vi "ProdaNG.Oracle.FindPath.vi"(8 "error in (no error)":errorcluster) -> (0 "error out":errorcluster, 1 "found":bool, 2 "Tnsnames path":path)   [LabVIEW 2016]
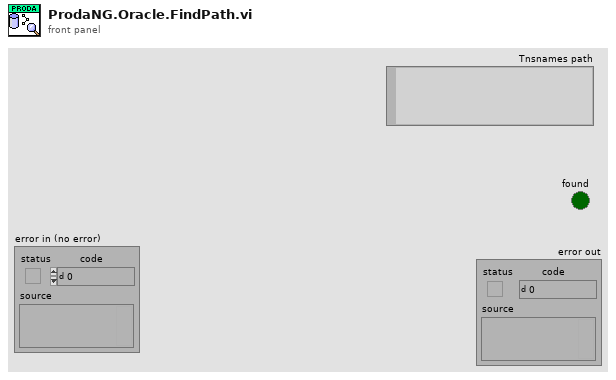
[diagram p1: front panel]
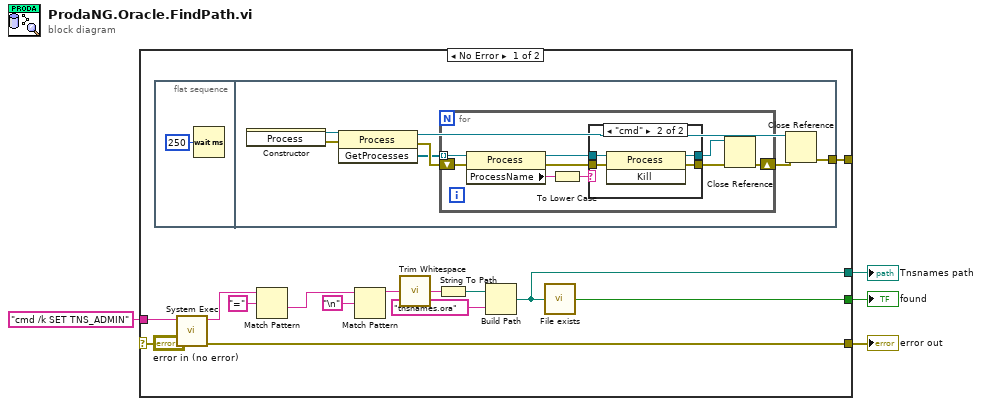
[diagram p0: block diagram]
diagram:
  n1 = case shown="No Error" "error in (no error)" {
    selector: "error in (no error)" -> [w18 w43]
    tunnel: "cmd /k SET TNS_ADMIN" ("command line") -> [w19 _]
    tunnel: [w17 w43] -> w4
    tunnel: [w11 _] -> w2
    tunnel: [w10 _] -> w1
    tunnel: [w6 _] -> _
    frame No Error {
      n2 = flat-sequence {
        tunnel: [w21] -> w6
        frame #0 {
          n3 = Wait (ms)(milliseconds to wait=u32 250) -> ()  [unwired: 1 out]
        }
        frame #1 {
          n4 = constructor class="Process"() -> (reference out=w27:refnum<k24>, error out=w26:errorcluster)  [unwired: 3 in, 1 out]
          n5 = invoke class="Process" method="GetProcesses"(reference=w27, error in=w26) -> (reference out=w22:refnum<k24>, error out=w25:errorcluster, "GetProcesses"=w24:refnum<k24>[])  [unwired: 1 in]
          n6 = for {
            tunnel: w24 -> [w36] mode=indexing
            shift-right: [w30] -> w23
            shift-left: w25 -> [w35]
            n7 = property class="Process"(reference=w36, error in=w35) -> (reference out=w34:refnum<k24>, error out=w33:errorcluster, "ProcessName"=w29:string)
            n8 = To Lower Case(string=w29) -> (all lower case string=w28:string)
            n9 = case shown="\"cmd\"" w28 {
              tunnel: w34 -> [w38 w42]
              tunnel: w33 -> [w37 w41]
              tunnel: [w37 w40] -> w32
              tunnel: [w38 w39] -> w31
              frame Default {
              }
              frame "cmd" {
                n10 = invoke class="Process" method="Kill"(reference=w42, error in=w41) -> (reference out=w39:refnum<k24>, error out=w40:errorcluster)  [unwired: 1 in, 1 out]
              }
            }
            n11 = Close Reference(reference=w31, error in (no error)=w32) -> (error out=w30:errorcluster)
          }
          n12 = Close Reference(reference=w22, error in (no error)=w23) -> (error out=w21:errorcluster)
        }
      }
      n13 = call <vilib>:"System Exec.vi"("error in (no error)"=w18, "command line"=w19) -> ("error out"=w17:errorcluster, "standard output"=w9:string)  [unwired: 6 in, 2 out]
      n14 = Match Pattern(string=w9, regular expression="=") -> (after substring=w7:string)  [unwired: 1 in, 3 out]
      n15 = Match Pattern(string=w7, regular expression="\n") -> (before substring=w15:string)  [unwired: 1 in, 3 out]
      n16 = call <vilib>:"Trim Whitespace.vi"("string"=w15) -> ("trimmed string"=w14:string)  [unwired: 1 in]
      n17 = String To Path(string=w14) -> (path=w13:path)
      n18 = Build Path(base path=w13, name or relative path="tnsnames.ora") -> (appended path=w11:path)
      n19 = call "File exists.vi"("file path"=w11) -> ("exists?"=w10:bool)  [unwired: 4 in]
    }
    frame Error {
    }
  }
  "error out" <- w4
  "found" <- w1
  "Tnsnames path" <- w2
